vi "Multi-Device_Sync-AI_and_AO-Shared_Timebase_&_Trig-DSA-PRI.vi"(10 "Samples per Channel":i32=20000 caption="Samples to Read per Loop", 11 "SampClk.Rate":dbl=150000.0) -> (3 "AO - AI":dbl=0.10014500617980959)   [LabVIEW 2019]
doc: "I. Description:\nThis example configures a total of four tasks on two PXI Dynamic Signal Acquistion (DSA) devices. Each device runs a task for analog input and another for analog output. This VI illustrates continuous analog input and ouptut operations.\n\nII. Instructions for Running:\n1. Select which type of Syncrhonization method you want to use.\n2. Select the physical channels to corresponding to the signal connection on each device.\n3. Enter the minimum and maximum expected voltage for the input and output operations on each device.\nNote: For optimal accuracy, match the input range to the expected voltage level of the measured signal (for input) and generated signal (for output).\n4. Set the number of samples to acquire per channel. This parameter determines how many points will be read and generated with each iteration of the WHILE loop.\n5. Set the rate of the acquisition and generation. The same sampling rate is employed for input and output operations on each device.\nNote: The sampling rate should be at least 2.2 times the maximum frequency component of the signal being acquired on analog input and the signal being generated on analog output. Frequency components beyond about 0.47 times the sampling rate will be eliminated by the alias and imaging protection on the DSA device.\n\nIII. Block Diagram Steps:\n1. Create an analog input and output channel for both the master and slave devices.\n2. Set timing parameters for a continuous acquisition. The sample rate and block size are set to the same values for each device.\n3. There are two types of synchronization available on DSA devices. The first method shares the Sample Clock Timebase across the PXI_Star bus. It also uses the Sync Pulse which is shared across the PXI_Trig / RTSI bus. The second method uses the Sync Pulse in conjunction with the PXI Reference clock 10 on the PXI backplane. \n4. Call the Get Terminal Name with Device Prefix VI to append the device name to the signal name for the acquisition start trigger. This signal is then used as an output generation trigger on the master as well as and acquisition start trigger and generation start trigger on the slave. The signal is shared along the PXI_Trig / RTSI bus.\n5. Synthesize a standard waveform (sine, square, or triangle) and load this data into the output RAM buffer for each device.\n6. Call the Start VI to start the acquisition and generation tasks. (Note: The flat case structure provides flow control so that the slave device is armed before the master so that the slave device does not miss the trigger.)\n7. Read all of the waveform data from both devices.\n8. Check the status of the analog output tasks on both devices.\n9. Call the Clear Task VI to stop the acquisition and generation and clear the task.\n10. Use the popup dialog box to display an error if any.\n\nIV. I/O Connections Overview:\nMake sure your signal input and output terminals matches the Physical Channel I/O controls.\n\nIt is important to ensure that your PXI chassis has been properly configured in MAX. If your chassis has not been configured in software before running the VI, your devices may fail to synchronize properly."
uses:
  <vilib>/Utility/error.llb/DialogType.ctl
  <vilib>/DAQmx/write.llb/DAQmx Write (Analog Wfm 1Chan NSamp).vi
  <vilib>/DAQmx/read.llb/DAQmx Read (Analog Wfm 1Chan NSamp).vi
  <vilib>/DAQmx/create/channels.llb/DAQmx Create Channel (AO-Voltage-Basic).vi
  <vilib>/DAQmx/configure/timing.llb/DAQmx Timing (Sample Clock).vi
  <vilib>/DAQmx/create/channels.llb/DAQmx Create Channel (AI-Voltage-Basic).vi
  <vilib>/DAQmx/configure/trigger.llb/DAQmx Start Trigger (Digital Edge).vi
  <vilib>/DAQmx/miscellaneous.llb/DAQmx Fill In Error Info.vi
  <resource>/objmgr/daqmx.rc
  Instrument.DAQ/Instrument.DAQ.lvclass
panel:
  out "AO time":dbl
  out "AO time 2":dbl
  out "AI time":dbl
  out "Input.OnbrdBufSize":u32
  out "Input.BufSize":u32
  out "Output.OnbrdBufSize":u32
  out "Output.BufSize":u32
  in  "RegenMode":i32(ring)=10158 items=["Allow Regeneration"=10097, "Do Not Allow Regeneration"=10158]
  out "Chart":dbl(graph)
  in  "Minimum Value":dbl=-10.0 caption="Output Minimum Value" format="%0.2f"
  in  "Maximum Value":dbl=10.0 caption="Output Maximum Value" format="%0.2f"
  in  "Physical Channel":tag="PXI1Slot3/ao0" caption="Master Output Physical Channels"
  in  "Maximum Value":dbl=10.0 caption="Input Maximum Value" format="%0.2f"
  in  "Minimum Value":dbl=-10.0 caption="Input Minimum Value" format="%0.2f"
  in  "Physical Channel":tag="PXI1Slot3/ai0" caption="Master Input Physical Channel"
  in  "stop":bool
  out "Measurement":waveform(dbl)[](graph)=[{"t0"=timestamp(0 s since 1904-01-01), "dt"=6.666666665308488e-06, "Y"=array[20000 elements]}, {"t0"=timestamp(3841587749.2572894 s since 1904-01-01), "dt"=6.666666665308468e-06, "Y"=array[20000 elements], "attributes"=variant("NI_ChannelName"=variant(string "PXI1Slot3/ai0"), "NI_UnitDescription"=variant(string "Volts"))}] caption="Measurement:  Master Board"
  # "For instructions, select Help>>Show Context Help"
  # "Channel Parameters:  Master Board"
  # "Timing Parameters"
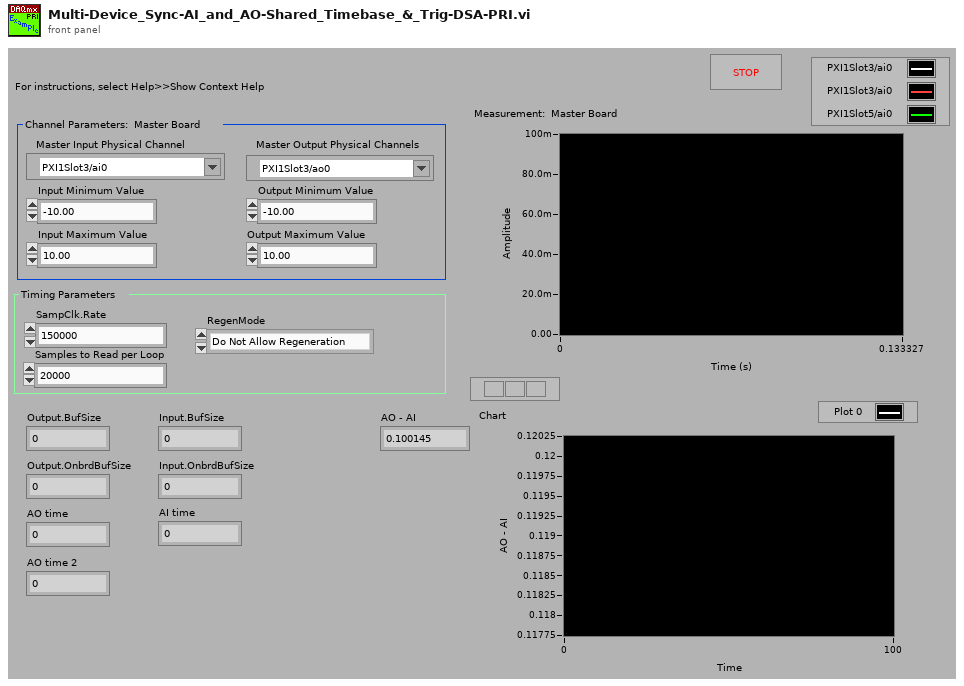
[diagram p1: front panel]
types:
  T1 = typedef "DialogType.ctl" = u16
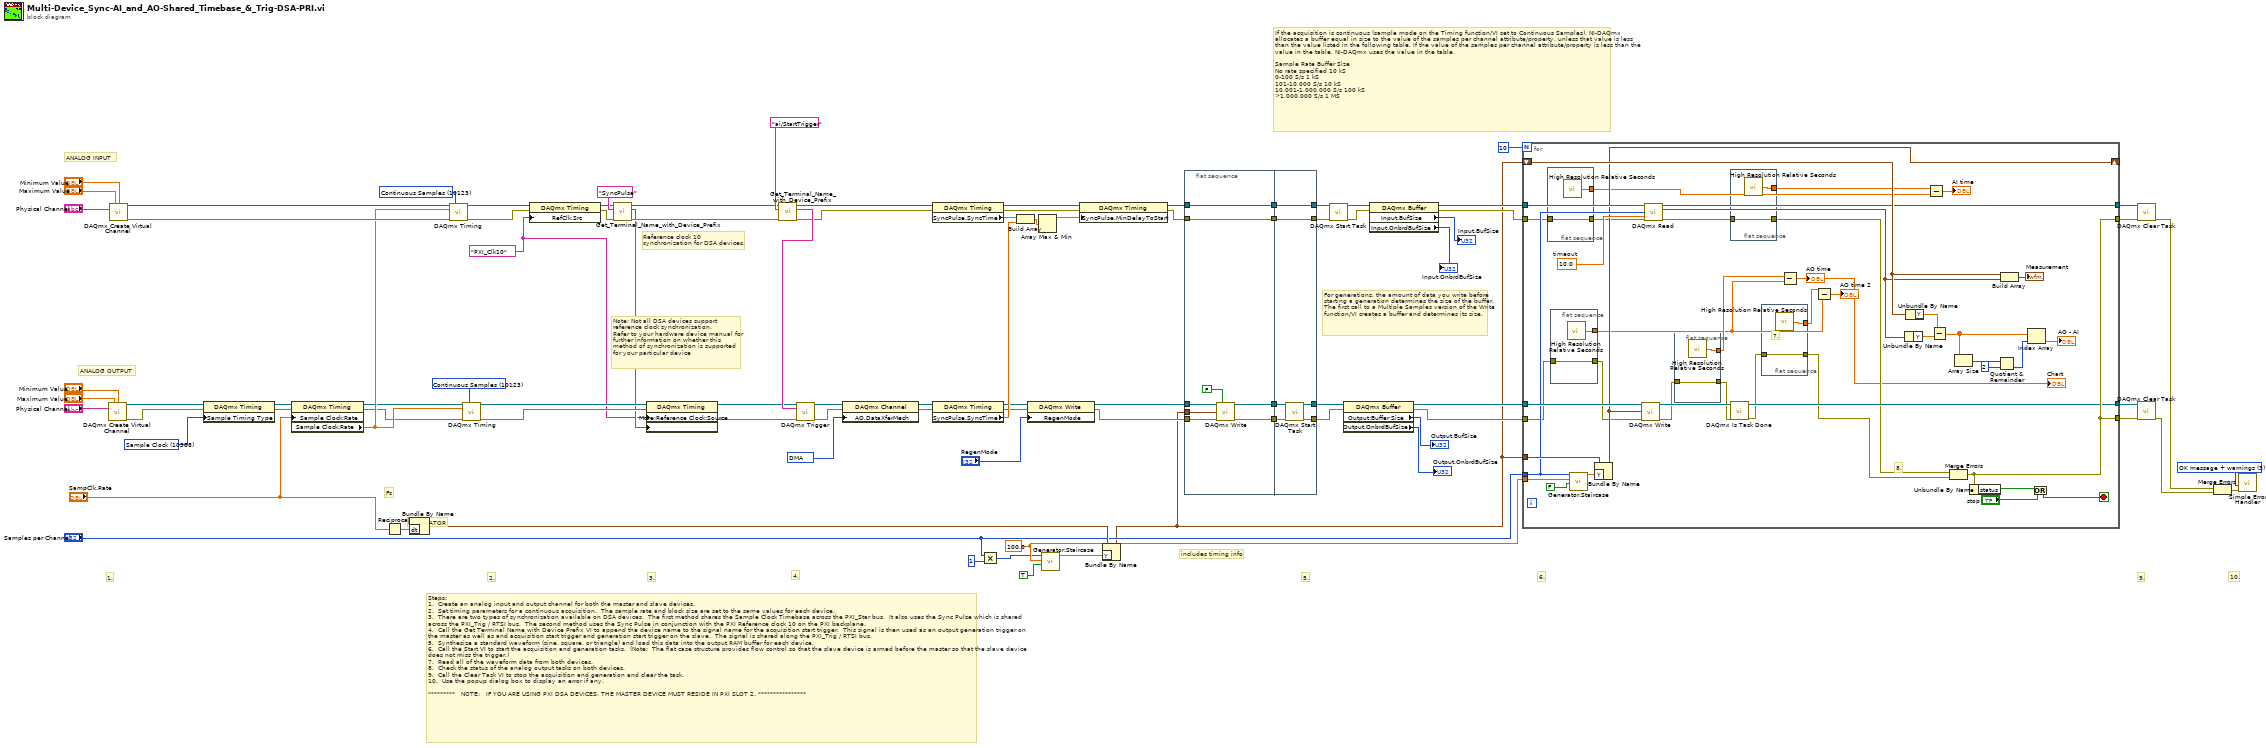
[diagram p0: block diagram]
diagram:
  w7 = 10054 items=["DMA"=10054, "Interrupts"=10204, "Programmed I/O"=10264, "USB Bulk"=12590] ("AO.DataXferMech")
  w13 = 10388 items=["Sample Clock"=10388, "Handshake"=10389, "Implicit"=10451, "On Demand"=10390, "Change Detection"=12504] ("SampTimingType")
  w23 = 10123 items=["Finite Samples"=10178, "Continuous Samples"=10123] ("sample mode")
  w42 = tag "PXI_Clk10" ("RefClk.Src")
  w54 = 100.0 ("period")
  w77 = T1 3 items=["no dialog", "OK message", "continue or stop message", "OK message + warnings", "continue/stop + warnings"] ("type of dialog (OK msg:1)")
  w86 = 10123 items=["Finite Samples"=10178, "Continuous Samples"=10123] ("sample mode")
  # "ANALOG OUTPUT"
  # "For generations, the amount of data you write before starting a generation determines the size of the buffer. The first call to a Multiple Samples version of the Write function/VI creates a buffer and determines its size."
  # "If the acquisition is continuous (sample mode on the Timing function/VI set to Continuous Samples), NI-DAQmx allocates a buffer equal in size to the value of the samples per channel attribute/property, unless that value is less than the value listed in the following table. If the value of the samples per channel attribute/property is less than the value in the table, NI-DAQmx uses the value in the table.\n\nSample Rate\tBuffer Size\nNo rate specified\t10 kS\n0-100 S/s\t1 kS\n101-10,000 S/s\t10 kS\n10,001-1,000,000 S/s\t100 kS\n>1,000,000 S/s\t1 MS"
  # "Fs"
  # "GENERATOR"
  # "ANALOG INPUT"
  # "Note: Not all DSA devices support\nreference clock synchronization.\nRefer to your hardware device manual for\nfurther information on whether this \nmethod of synchronization is supported\nfor your particular device"
  # "Reference clock 10\nsynchronization for DSA devices."
  # "includes timing info"
  # "10."
  # "9."
  # "Steps: \n1.  Create an analog input and output channel for both the master and slave devices.\n2.  Set timing parameters for a continuous acquisition.  The sample rate and block size are set to the same values for each device.\n3.  There are two types of synchronization available on DSA devices.  The first method shares the Sample Clock Timebase across the PXI_Star bus.  It also uses the Sync Pulse which is shared across the PXI_Trig / RTSI bus.  The second method uses the Sync Pulse in conjunction with the PXI Reference clock 10 on the PXI backplane. \n4.  Call the Get Terminal Name with Device Prefix VI to append the device name to the signal name for the acquisition start trigger.  This signal is then used as an output generation trigger on the master as well as and acquisition start trigger and generation start trigger on the slave.  The signal is shared along the PXI_Trig / RTSI bus.\n5.  Synthesize a standard waveform (sine, square, or triangle) and load this data into the output RAM buffer for each device.\n6.  Call the Start VI to start the acquisition and generation tasks.  (Note:  The flat case structure provides flow control so that the slave device is armed before the master so that the slave device does not miss the trigger.)\n7.  Read all of the waveform data from both devices.\n8.  Check the status of the analog output tasks on both devices.\n9.  Call the Clear Task VI to stop the acquisition and generation and clear the task.\n10.  Use the popup dialog box to display an error if any.\n\n*********   NOTE:  \tIF YOU ARE USING PXI DSA DEVICES, THE MASTER DEVICE MUST RESIDE IN PXI SLOT 2. ****************"
  # "6."
  # "5."
  # "4."
  # "3."
  # "2."
  # "1."
  n1 = call-poly <vilib>:"DAQmx Create Virtual Channel.vi"("maximum value"="Maximum Value", "minimum value"="Minimum Value", "physical channels"="Physical Channel") -> ("task out"=w19:refnum<k21>, "error out"=w14:errorcluster)  [unwired: 11 in]
  n2 = call-poly <vilib>:"DAQmx Create Virtual Channel.vi"("maximum value"="Maximum Value", "minimum value"="Minimum Value", "physical channels"="Physical Channel") -> ("task out"=w88:refnum<k21>, "error out"=w90:errorcluster)  [unwired: 11 in]
  n3 = property class="DAQmx Timing"(reference=w19, error in=w14, "Sample Timing Type"=w13) -> (reference out=w15:refnum<k21>, error out=w16:errorcluster)
  n4 = property class="DAQmx Timing"(reference=w15, error in=w16, "Sample Clock:Rate"="SampClk.Rate") -> (reference out=w17:refnum<k21>, error out=w18:errorcluster, "Sample Clock:Rate"=w26:dbl)
  n5 = Reciprocal(x="SampClk.Rate") -> (1/x=w48:dbl)
  n6 = Bundle By Name("dt"=w48) -> (w47:waveform(dbl))  [unwired: 1 in]
  n7 = call-poly <vilib>:"DAQmx Timing.vi"("task/channels in"=w88, "sample mode"=w86, "rate"=w26, "error in"=w90) -> ("task out"=w85:refnum<k21>, "error out"=w84:errorcluster)  [unwired: 10 in]
  n8 = call-poly <vilib>:"DAQmx Timing.vi"("task/channels in"=w17, "sample mode"=w23, "rate"=w26, "error in"=w18) -> ("task out"=w76:refnum<k21>, "error out"=w75:errorcluster)  [unwired: 10 in]
  n9 = property class="DAQmx Timing"(reference=w85, error in=w84, "RefClk.Src"=w42) -> (reference out=w43:refnum<k21>, error out=w41:errorcluster)
  n10 = call "Get_Terminal_Name_with_Device_Prefix.vi"("error in (no error)"=w41, "Local Terminal Name"="SyncPulse", "task/channels in"=w43) -> ("error out"=w70:errorcluster, "Terminal Name with Device Prefix"=w44:tag, "task out"=w71:refnum<k21>)  [unwired: 6 in]
  n11 = property class="DAQmx Timing"(reference=w76, error in=w75, "More:Reference Clock:Source"=w42, "More:Synchronization Pulse:Source"=w44) -> (reference out=w12:refnum<k21>, error out=w11:errorcluster)
  n12 = call "Get_Terminal_Name_with_Device_Prefix.vi"("error in (no error)"=w70, "Local Terminal Name"="ai/StartTrigger", "task/channels in"=w71) -> ("error out"=w67:errorcluster, "Terminal Name with Device Prefix"=w69:tag, "task out"=w68:refnum<k21>)  [unwired: 6 in]
  n13 = call-poly <vilib>:"DAQmx Trigger.vi"("task/channels in"=w12, "source"=w69, "error in"=w11) -> ("task out"=w6:refnum<k21>, "error out"=w3:errorcluster)  [unwired: 11 in]
  n14 = property class="DAQmx Channel"(reference=w6, error in=w3, "AO.DataXferMech"=w7) -> (reference out=w5:refnum<k21>, error out=w4:errorcluster)
  n15 = property class="DAQmx Timing"(reference=w68, error in=w67) -> (reference out=w53:refnum<k21>, error out=w66:errorcluster, "SyncPulse.SyncTime"=w24:dbl)
  n16 = property class="DAQmx Timing"(reference=w5, error in=w4) -> (reference out=w9:refnum<k21>, error out=w8:errorcluster, "SyncPulse.SyncTime"=w25:dbl)
  n17 = Multiply(x="Samples per Channel", y=1) -> (x*y=w49:i32)
  n18 = Build Array(w24, w25) -> (w65:dbl[])
  n19 = property class="DAQmx Write"(reference=w9, error in=w8, "RegenMode"="RegenMode") -> (reference out=w40:refnum<k21>, error out=w39:errorcluster)
  n20 = Array Max & Min(array=w65) -> (max value=w64:dbl)  [unwired: 3 out]
  n21 = call "Generator.Staircase.vi"("reset?"=TRUE, "period"=w54, "dimension size"=w49) -> ("Array"=w57:dbl[])  [unwired: 8 in]
  n22 = property class="DAQmx Timing"(reference=w53, error in=w66, "SyncPulse.MinDelayToStart"=w64) -> (reference out=w62:refnum<k21>, error out=w63:errorcluster)
  n23 = Bundle By Name(cluster=w47, "Y"=w57) -> (w29:waveform(dbl))
  n24 = flat-sequence {
    tunnel: [w98] -> w61
    tunnel: [w97] -> w60
    tunnel: [w94] -> w59
    tunnel: [w93] -> w58
    tunnel: w29 -> [w92]
    tunnel: w62 -> [w98]
    tunnel: w63 -> [w97]
    tunnel: w39 -> [w96]
    tunnel: w40 -> [w95]
    tunnel: [w103] -> w38
    tunnel: [w104] -> w37
    tunnel: [w102] -> w74
    tunnel: [w101] -> w73
    tunnel: w61 -> [w102]
    tunnel: w60 -> [w101]
    tunnel: w59 -> [w100]
    tunnel: w58 -> [w99]
    frame #0 {
      n25 = call-poly <vilib>:"DAQmx Write.vi"("task/channels in"=w95, "auto start"=FALSE, "data"=w92, "error in"=w96) -> ("task out"=w93:refnum<k21>, "error out"=w94:errorcluster)  [unwired: 9 in, 1 out]
    }
    frame #1 {
      n26 = call <vilib>:"DAQmx Start Task.vi"("task/channels in"=w99, "error in"=w100) -> ("task out"=w104:refnum<k21>, "error out"=w103:errorcluster)  [unwired: 12 in]
    }
  }
  n27 = call <vilib>:"DAQmx Start Task.vi"("task/channels in"=w74, "error in"=w73) -> ("task out"=w31:refnum<k21>, "error out"=w30:errorcluster)  [unwired: 12 in]
  n28 = property class="DAQmx Buffer"(reference=w37, error in=w38) -> (reference out=w36:refnum<k21>, error out=w35:errorcluster, "Output:Buffer Size"=→"Output.BufSize":u32, "Output.OnbrdBufSize"=→"Output.OnbrdBufSize":u32)
  n29 = property class="DAQmx Buffer"(reference=w31, error in=w30) -> (reference out=w33:refnum<k21>, error out=w32:errorcluster, "Input.BufSize"=→"Input.BufSize":u32, "Input.OnbrdBufSize"=→"Input.OnbrdBufSize":u32)
  n30 = for {
    N: 10 -> [_]
    tunnel: [w146] -> w89
    tunnel: w33 -> [w139]
    tunnel: [w124] -> w87
    tunnel: w36 -> [w145]
    tunnel: w32 -> [w122]
    tunnel: [w125] -> w83
    tunnel: [w146] -> w82
    tunnel: w35 -> [w115]
    tunnel: w29 -> [w144]
    tunnel: "Samples per Channel" -> [w134]
    tunnel: w54 -> [w140]
    shift-right: [w132] -> _
    shift-left: w29 -> [w133]
    stop <- w141 stop-if-true
    w137 = 10.0  # timeout
    # "8."
    # "7."
    n31 = flat-sequence {
      tunnel: [w156] -> w123
      tunnel: w122 -> [w156]
      tunnel: [w155] -> w118
      frame #0 {
        n32 = call <vilib>:"High Resolution Relative Seconds.vi"() -> ("relative seconds"=w155:dbl)
      }
    }
    n33 = flat-sequence {
      tunnel: [w152] -> w114
      tunnel: w115 -> [w152]
      tunnel: [w151] -> w106
      frame #0 {
        n34 = call <vilib>:"High Resolution Relative Seconds.vi"() -> ("relative seconds"=w151:dbl)
      }
    }
    n35 = call "Generator.Staircase.vi"("reset?"=FALSE, "period"=w140, "dimension size"=w134) -> ("Array"=w136:dbl[])  [unwired: 8 in]
    n36 = Bundle By Name(cluster=w144, "Y"=w136) -> (w132:waveform(dbl))
    n37 = call-poly <vilib>:"DAQmx Write.vi"("task/channels in"=w145, "data"=w132, "error in"=w114) -> ("task out"=w116:refnum<k21>, "error out"=w109:errorcluster)  [unwired: 10 in, 1 out]
    n38 = call-poly <vilib>:"DAQmx Read.vi"("task/channels in"=w139, "number of samples per channel"=w134, "timeout"=w137, "error in"=w123) -> ("task out"=w124:refnum<k21>, "data"=w130:waveform(dbl), "error out"=w121:errorcluster)  [unwired: 9 in]
    n39 = flat-sequence {
      tunnel: w109 -> [w150]
      tunnel: [w150] -> w108
      tunnel: [w149] -> w107
      frame #0 {
        n40 = call <vilib>:"High Resolution Relative Seconds.vi"() -> ("relative seconds"=w149:dbl)
      }
    }
    n41 = flat-sequence {
      tunnel: w121 -> [w158]
      tunnel: [w158] -> w120
      tunnel: [w157] -> w119
      frame #0 {
        n42 = call <vilib>:"High Resolution Relative Seconds.vi"() -> ("relative seconds"=w157:dbl)
      }
    }
    n43 = call <vilib>:"DAQmx Is Task Done.vi"("task/channels in"=w116, "error in"=w108) -> ("task out"=w125:refnum<k21>, "error out"=w113:errorcluster)  [unwired: 11 in, 1 out]
    n44 = flat-sequence {
      tunnel: w113 -> [w154]
      tunnel: [w154] -> w112
      tunnel: [w153] -> w110
      frame #0 {
        n45 = call <vilib>:"High Resolution Relative Seconds.vi"() -> ("relative seconds"=w153:dbl)
      }
    }
    n46 = Subtract(x=w107, y=w106) -> (x-y=→"Chart" →"AO time":dbl)
    n47 = Subtract(x=w110, y=w106) -> (x-y=→"AO time 2":dbl)
    n48 = Unbundle By Name(w130) -> ("Y"=w131:dbl[])
    n49 = Unbundle By Name(w133) -> ("Y"=w129:dbl[])
    n50 = Subtract(x=w119, y=w118) -> (x-y=→"AI time":dbl)
    n51 = Subtract(x=w129, y=w131) -> (x-y=w128:dbl[])
    n52 = Merge Errors(w120, w112) -> (w146:errorcluster)
    n53 = Array Size(array=w128) -> (size(s)=w138:i32)
    n54 = Unbundle By Name(w146) -> ("status"=w148:bool)
    n55 = Quotient & Remainder(x=w138, y=2) -> (floor(x/y)=w127:i32)  [unwired: 1 out]
    n56 = Build Array(w133, w130) -> (→"Measurement":waveform(dbl)[])
    n57 = Index Array(array=w128, index=w127) -> (element=→"AO - AI":dbl)
    n58 = Or(x=w148, y="stop") -> (x .or. y?=w141:bool)
  }
  n59 = call <vilib>:"DAQmx Clear Task.vi"("task in"=w87, "error in"=w89) -> ("error out"=w52:errorcluster)  [unwired: 13 in]
  n60 = call <vilib>:"DAQmx Clear Task.vi"("task in"=w83, "error in"=w82) -> ("error out"=w51:errorcluster)  [unwired: 13 in]
  n61 = Merge Errors(w52, w51) -> (w81:errorcluster)
  n62 = call <vilib>:"Simple Error Handler.vi"("type of dialog (OK msg:1)"=w77, "error in (no error)"=w81) -> ()  [unwired: 3 in, 5 out]
